vi "Loop_SEN.vi"() -> ()   [LabVIEW 2017, in "Dashboard.lvlib"]
uses:
  Dashboard.lvlib
  _SHARE ALL/Global Share All/Global_STOP.vi
panel:
  out "Cycle Time (S)":dbl format="%.3g"
  in  "Target Time(ms)":u32=50
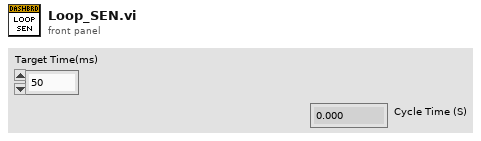
[diagram p1: front panel]
types:
  T1 = cluster{"Target Time(ms)":u32, "Current Time":timestamp, "Previous Time":timestamp, "Cycle Time (S)":dbl, "Num NET Vars":i32}
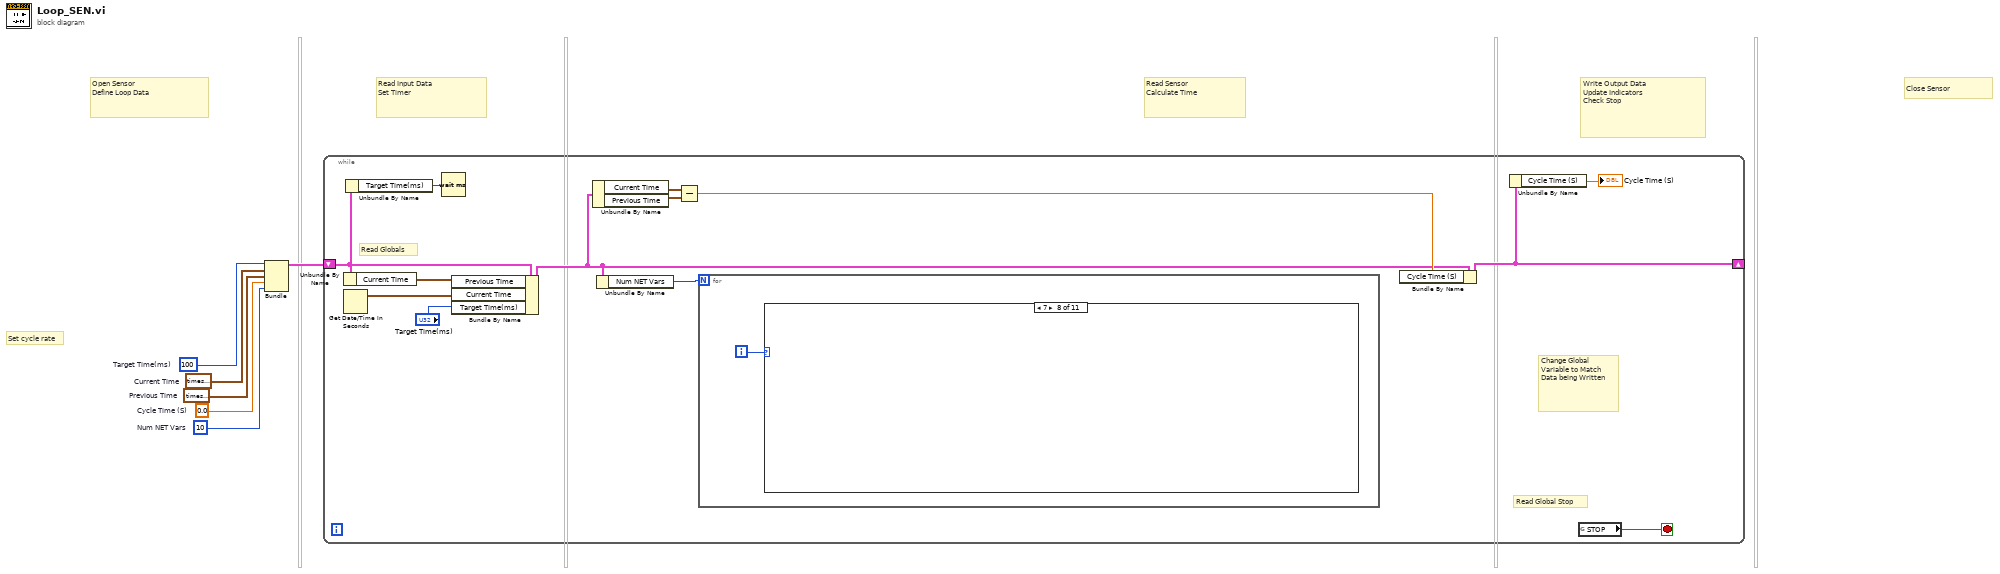
[diagram p0: block diagram]
diagram:
  w1 = 10  # Num NET Vars
  w2 = 0.0  # Cycle Time (S)
  w6 = timestamp(0 s since 1904-01-01)  # Previous Time
  w5 = timestamp(0 s since 1904-01-01)  # Current Time
  w4 = u32 100  # Target Time(ms)
  # "Close Sensor"
  # "Write Output Data\nUpdate Indicators\nCheck Stop"
  # "Read Sensor\nCalculate Time"
  # "Read Input Data\nSet Timer"
  # "Open Sensor\nDefine Loop Data"
  # "Set cycle rate"
  n1 = Bundle("Target Time(ms)"=w4, "Current Time"=w5, "Previous Time"=w6, "Cycle Time (S)"=w2, "Num NET Vars"=w1) -> (w3:T1)  [unwired: 1 in]
  n2 = while {
    shift-right: [w11] -> _
    shift-left: w3 -> [w13]
    stop <- w19 stop-if-true
    # "Change Global\nVariable to Match\nData being Written"
    # "Read Globals"
    # "Read Global Stop"
    n3 = Unbundle By Name(w13) -> ("Current Time"=w17:timestamp)
    n4 = Get Date/Time In Seconds() -> (seconds since 1Jan1904=w18:timestamp)
    n5 = Unbundle By Name(w13) -> ("Target Time(ms)"=w12:u32)
    n6 = Wait (ms)(milliseconds to wait=w12) -> ()  [unwired: 1 out]
    n7 = Bundle By Name(cluster=w13, "Previous Time"=w17, "Current Time"=w18, "Target Time(ms)"="Target Time(ms)") -> (w8:T1)
    n8 = Unbundle By Name(w8) -> ("Current Time"=w16:timestamp, "Previous Time"=w15:timestamp)
    n9 = Unbundle By Name(w8) -> ("Num NET Vars"=w7:i32)
    n10 = Subtract(x=w16, y=w15) -> (x-y=w9:dbl)
    n11 = for {
      N: w7 -> [_]
      i -> [w20]
      n12 = case shown="7" w20 {
        frame ..0 {
        }
        frame 1 {
        }
        frame 2 {
        }
        frame 3 {
        }
        frame 4 {
        }
        frame 5 {
        }
        frame 6 {
        }
        frame 7 {
        }
        frame 8 {
        }
        frame 9 {
        }
        frame 10.. {
        }
      }
    }
    n13 = Bundle By Name(cluster=w8, "Cycle Time (S)"=w9) -> (w11:T1)
    n14 = Unbundle By Name(w11) -> ("Cycle Time (S)"=→"Cycle Time (S)":dbl)
    n15 = global read "Global_STOP.vi" "STOP"() -> (w19:bool)
  }
